vi "Write LibraryDirectories.vi"(10 "LibraryDirectories":T1, 11 "ProjectItem in":refnum<class "Search.lvclass">) -> (3 "ProjectItem out":refnum<class "Search.lvclass">)   [LabVIEW 2016, in "Search.lvclass"]
uses:
  Search.lvclass
  Typedefs/LibraryDirectories.ctl
  Search.lvclass/Search.ctl
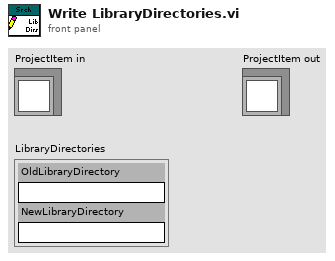
[diagram p1: front panel]
types:
  T1 = typedef "LibraryDirectories.ctl" = cluster{"OldLibraryDirectory":string, "NewLibraryDirectory":string}
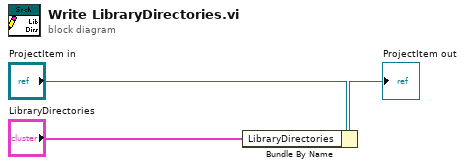
[diagram p0: block diagram]
diagram:
  n1 = Bundle By Name(cluster="ProjectItem in", "LibraryDirectories"="LibraryDirectories") -> (→"ProjectItem out":refnum<class "Search.lvclass">)
